vi "Read TempChamber.vi"(8 "error in (no error)":errorcluster, 11 "Execute in":refnum<class "Execute.lvclass">) -> (0 "error out":errorcluster, 2 "QMH_Class.lvlib:Device.lvlib:TempChamber Interface.lvclass":refnum<class "TempChamber Interface.lvclass">, 3 "Execute out":refnum<class "Execute.lvclass">)   [LabVIEW 2018, in "QMH_Class.lvlib" / "TestManager.lvlib" / "Execute.lvclass"]
uses:
  Execute.lvclass
  Device/TempChamber/TempChamber Interface/TempChamber Interface.lvclass
  Execute.lvclass/Execute.ctl
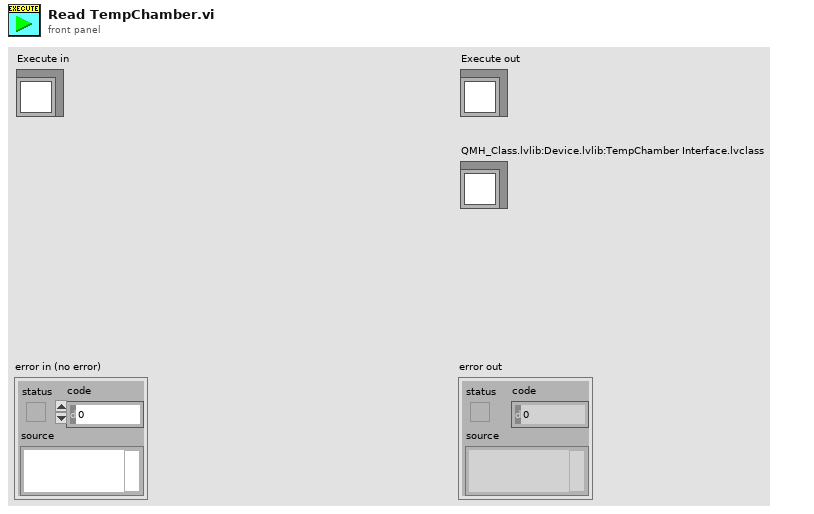
[diagram p1: front panel]
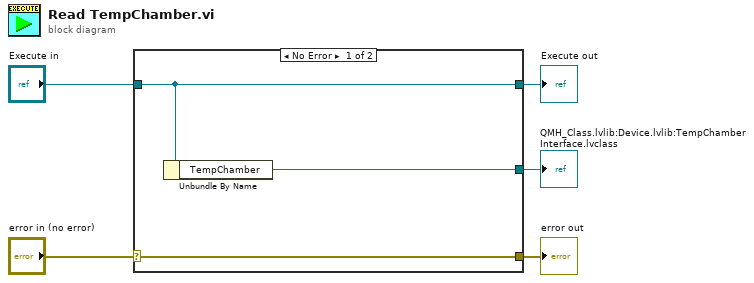
[diagram p0: block diagram]
diagram:
  n1 = case shown="No Error" "error in (no error)" {
    selector: "error in (no error)" -> [w8 w9]
    tunnel: [w8 w9] -> w4
    tunnel: [w7 w10] -> w2
    tunnel: "Execute in" -> [w7 w10]
    tunnel: [w6 _] -> w1
    frame No Error {
      n2 = Unbundle By Name(w7) -> ("TempChamber"=w6:refnum<class "TempChamber Interface.lvclass">)
    }
    frame Error {
    }
  }
  "error out" <- w4
  "Execute out" <- w2
  "QMH_Class.lvlib:Device.lvlib:TempChamber Interface.lvclass" <- w1
